vi "KMRmOS6RC Arm Control.vi"(8 "error in (no error)":errorcluster, 9 "clip":dbl(slide)=15.0 scale=0.0..15.0, 10 "turn":dbl(knob) scale=-150.0..110.0) -> (0 "error out":errorcluster, 1 "clipout":dbl, 2 "turnout":dbl)   [LabVIEW 2019]
uses:
  KNRm_ReMi_OS6_436Motor.lvlibp/KNRm_ReMi_Toolkit/IO/LowLevel/IO_Channel_RC.ctl
  math/Global 1.vi
  KNRm_ReMi_OS6_436Motor.lvlibp
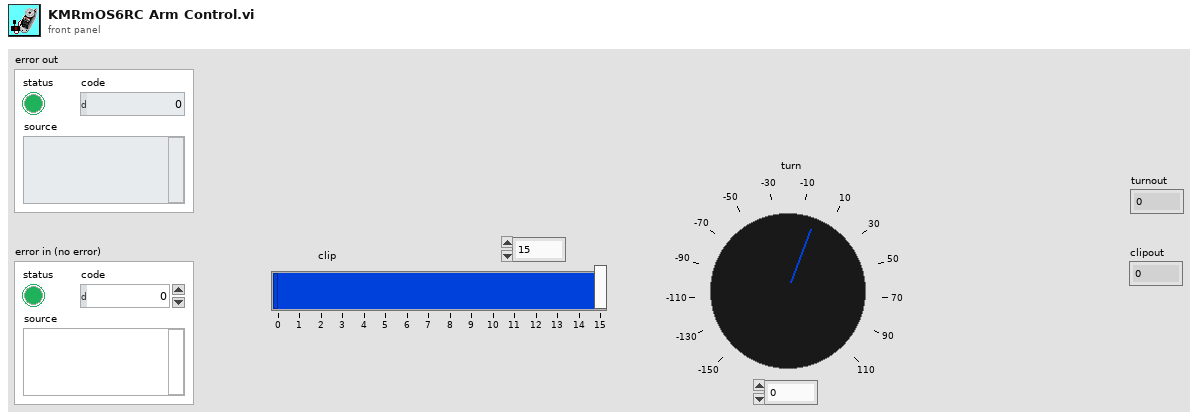
[diagram p1: front panel]
types:
  T1 = typedef "KNRm_ReMi_OS6_436Motor.lvlibp/IO_Channel_RC.ctl" = enum16{"RC1", "RC2", "S1(EXTIOB)", "S2(EXTIOB)", "S3(EXTIOB)", "S4(EXTIOB)", "S5(EXTIOB)", "S6(EXTIOB)"}
  T2 = cluster{"等比調整到角度正確":cluster{"S1":dbl, "S2":dbl, "S3":dbl, "S4":dbl, "S5":dbl}, "補償角度到0度是水平":cluster{"S1":dbl, "S2":dbl, "S3":dbl, "S4":dbl, "S5":dbl}}
  T3 = cluster{"S1":dbl, "S2":dbl, "S3":dbl, "S4":dbl, "S5":dbl}
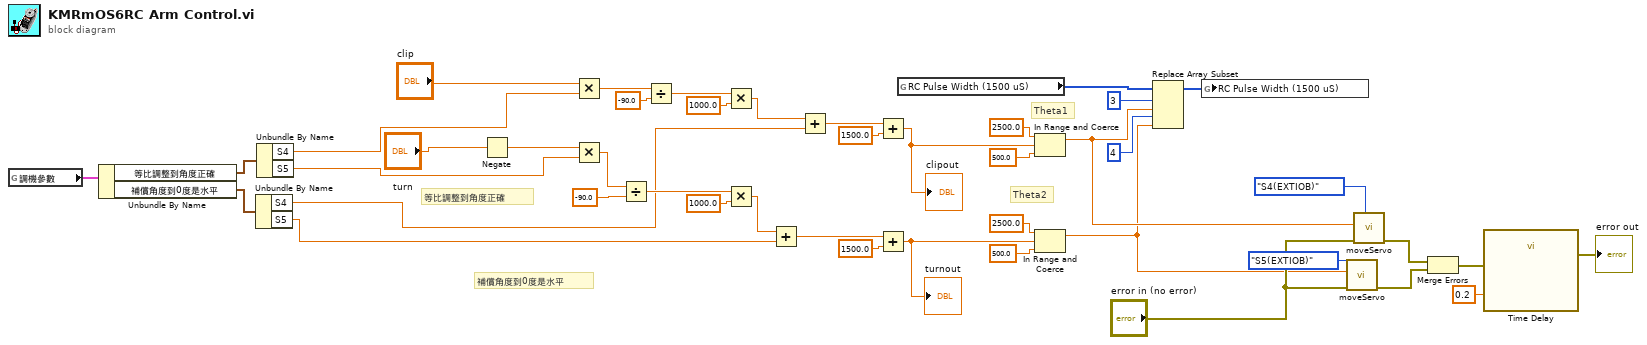
[diagram p0: block diagram]
diagram:
  # "補償角度到0度是水平"
  # "等比調整到角度正確"
  # "Theta2"
  # "Theta1"
  n1 = global read "Global 1.vi" "調機參數"() -> (w7:T2)
  n2 = Unbundle By Name(w7) -> ("等比調整到角度正確"=w5:T3, "補償角度到0度是水平"=w6:T3)
  n3 = Unbundle By Name(w6) -> ("S4"=w2:dbl, "S5"=w1:dbl)
  n4 = Unbundle By Name(w5) -> ("S4"=w4:dbl, "S5"=w3:dbl)
  n5 = Negate(x="turn") -> (-x=w30:dbl)
  n6 = Multiply(x="clip", y=w4) -> (x*y=w29:dbl)
  n7 = Multiply(x=w30, y=w3) -> (x*y=w28:dbl)
  n8 = Divide(x=w28, y=-90.0) -> (x/y=w37:dbl)
  n9 = Divide(x=w29, y=-90.0) -> (x/y=w41:dbl)
  n10 = Multiply(x=w41, y=1000.0) -> (x*y=w25:dbl)
  n11 = Multiply(x=w37, y=1000.0) -> (x*y=w27:dbl)
  n12 = Add(x=w27, y=w1) -> (x+y=w26:dbl)
  n13 = Add(x=w25, y=w2) -> (x+y=w24:dbl)
  n14 = Add(x=w24, y=1500.0) -> (x+y=w32:dbl)
  "clipout" <- w32
  n15 = Add(x=w26, y=1500.0) -> (x+y=w31:dbl)
  "turnout" <- w31
  n16 = global read "Global 1.vi" "RC Pulse Width (1500 uS)"() -> (w23:u16[])
  n17 = In Range and Coerce(upper limit=2500.0, x=w32, lower limit=500.0) -> (coerced(x)=w9:dbl)  [unwired: 1 out]
  n18 = In Range and Coerce(upper limit=2500.0, x=w31, lower limit=500.0) -> (coerced(x)=w8:dbl)  [unwired: 1 out]
  n19 = Replace Array Subset(array=w23, new element #1=w9, index #1=3 ("index"), new element #2=w8, index #2=4 ("index")) -> (w21:u16[])
  n20 = global write "Global 1.vi" "RC Pulse Width (1500 uS)"(w21) -> ()
  n21 = call "moveServo.vi"("Channel"=IO_Channel_RC."S5(EXTIOB)", "error in (no error)"="error in (no error)", "Servo Position (us)"=w8) -> ("error out"=w12:errorcluster)  [unwired: 8 in]
  n22 = call "moveServo.vi"("Channel"=IO_Channel_RC."S4(EXTIOB)", "error in (no error)"="error in (no error)", "Servo Position (us)"=w9) -> ("error out"=w13:errorcluster)  [unwired: 8 in]
  n23 = Merge Errors(w13, w12) -> (w11:errorcluster)
  n24 = call "Time Delay"("error in (no error)"=w11, "Delay Time (s)"=0.2) -> ("error out"=→"error out":errorcluster)  [unwired: 9 in]
